vi "Defer Panel Updates.vi"(8 "error in (no error)":errorcluster, 10 "Defer Panel Updates":bool, 11 "Graph Manager in":refnum<class "Graph Manager.lvclass">) -> (0 "error out":errorcluster, 3 "Graph Manager out":refnum<class "Graph Manager.lvclass">)   [LabVIEW 2016, in "Graph Manager.lvclass"]
uses:
  Graph Manager.lvclass
  Graph Manager.lvclass/Graph Manager.ctl
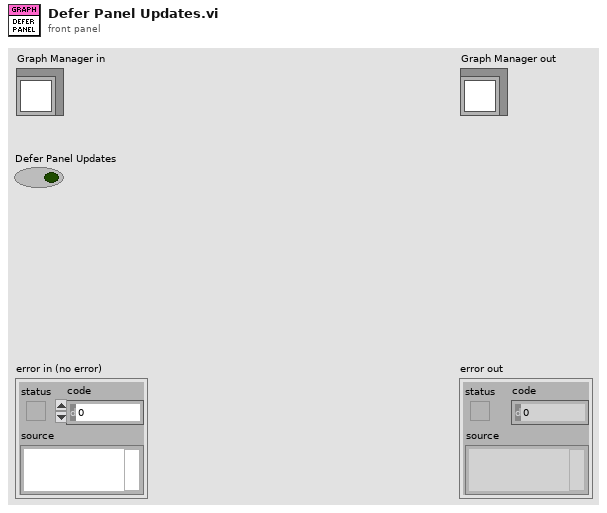
[diagram p1: front panel]
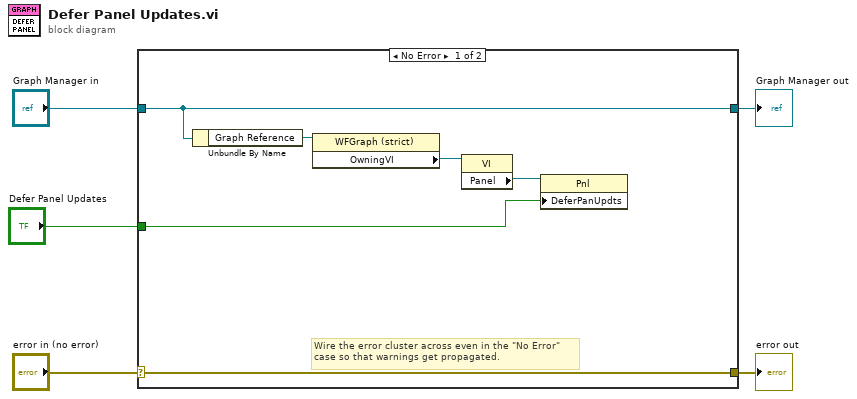
[diagram p0: block diagram]
diagram:
  n1 = case shown="No Error" "error in (no error)" {
    selector: "error in (no error)" -> [w11 w13]
    tunnel: [w11 w13] -> w4
    tunnel: [w10 w12] -> w2
    tunnel: "Graph Manager in" -> [w10 w12]
    tunnel: "Defer Panel Updates" -> [w6 _]
    frame No Error {
      # "Wire the error cluster across even in the \"No Error\"\ncase so that warnings get propagated."
      n2 = Unbundle By Name(w10) -> ("Graph Reference"=w9:refnum<vi>)
      n3 = property class="WFGraph (strict)"(reference=w9) -> ("OwningVI"=w8:refnum<vi>)  [unwired: 1 in, 2 out]
      n4 = property class="VI"(reference=w8) -> ("Panel"=w7:refnum<vi>)  [unwired: 1 in, 2 out]
      n5 = property class="Pnl"(reference=w7, "DeferPanUpdts"=w6) -> ()  [unwired: 1 in, 2 out]
    }
    frame Error {
    }
  }
  "error out" <- w4
  "Graph Manager out" <- w2
